vi "test notifier.vi"() -> ()   [LabVIEW 2019]
uses:
  Controls/FGV States.ctl
panel:
  in  "stop":bool
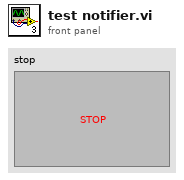
[diagram p1: front panel]
types:
  T1 = typedef "FGV States.ctl" = enum16{"Read", "Write"}
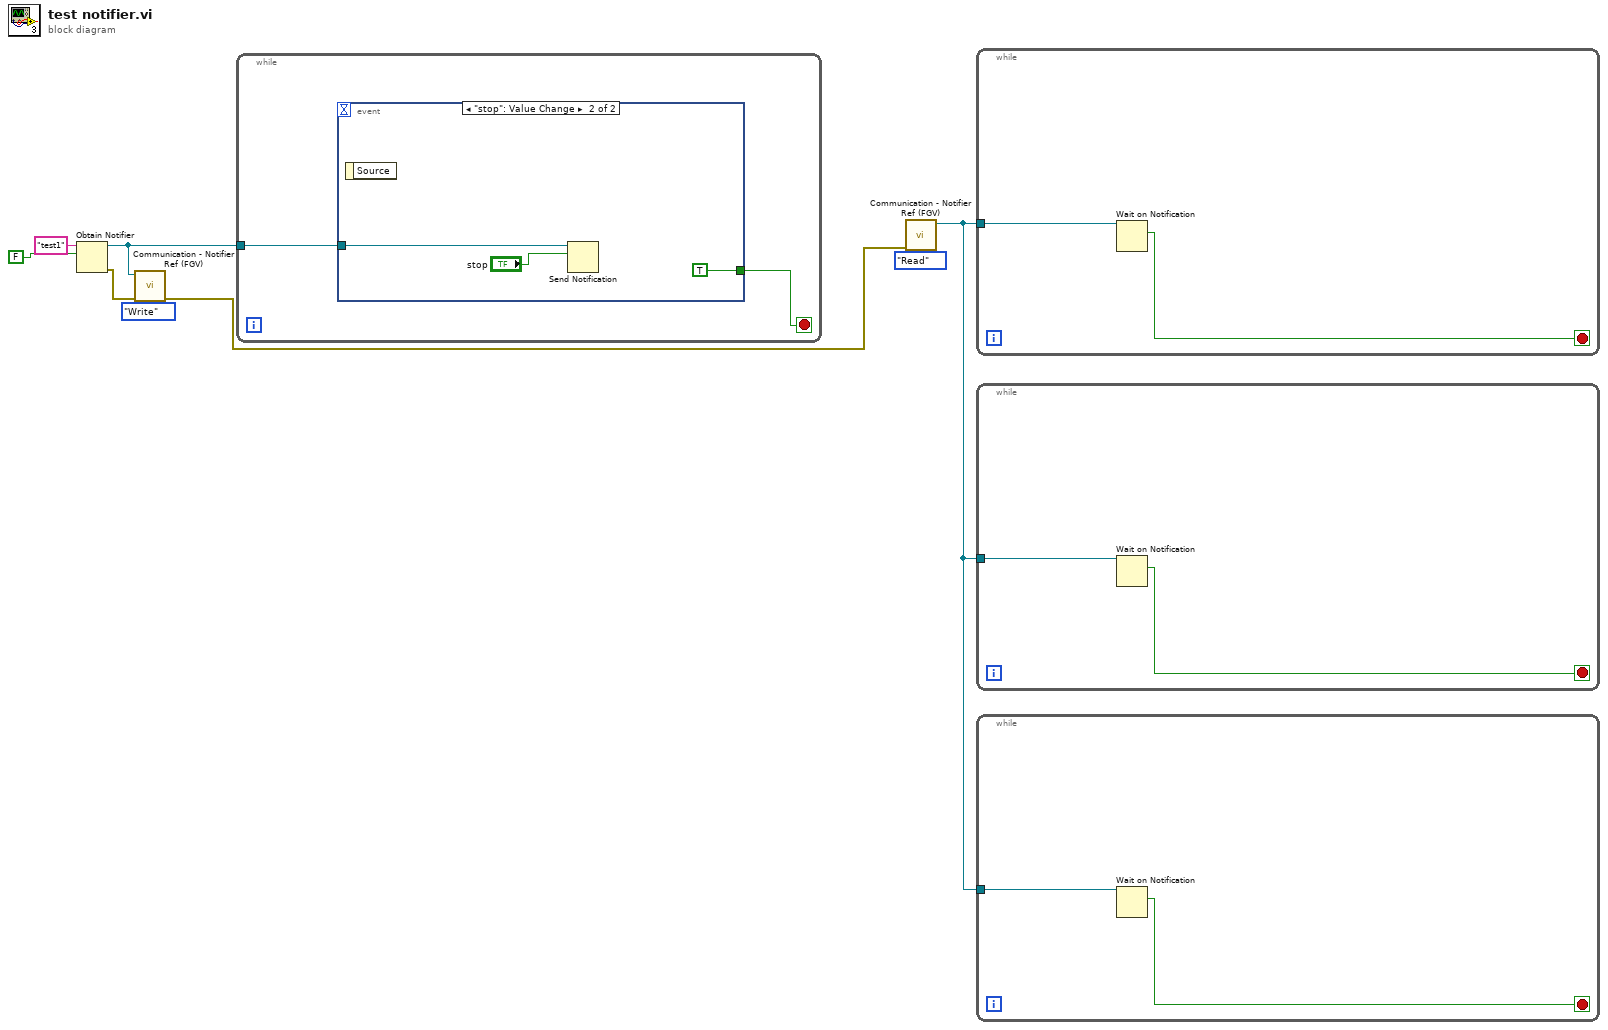
[diagram p0: block diagram]
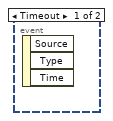
[diagram p2: hidden frame]
diagram:
  n1 = Obtain Notifier(name (unnamed)="test1", notification data type=FALSE) -> (notifier out=w6:refnum<notifier>, error out=w4:errorcluster)  [unwired: 2 in, 1 out]
  n2 = call "Communication - Notifier Ref (FGV).vi"("Action"=FGV_States."Write", "error in (no error)"=w4, "notifier in"=w6) -> ("error out"=w2:errorcluster)  [unwired: 7 in, 1 out]
  n3 = while {
    tunnel: w6 -> [w10]
    stop <- w9 stop-if-true
    n4 = event shown="[1] \"stop\": Value Change" {
      selector: _ -> [_ _]
      dyn-events: _ -> [_ _]
      timeout: _ -> [_ _]
      tunnel: w10 -> [_ w12]
      tunnel: [_ TRUE] -> w9
      event Timeout {
        n5 = event-data() -> ()  [unwired: 1 in, 3 out]
      }
      event "stop": Value Change {
        n6 = event-data() -> ()  [unwired: 1 in, 1 out]
        n7 = Send Notification(notification="stop", notifier=w12) -> ()  [unwired: 1 in, 2 out]
      }
    }
  }
  n8 = call "Communication - Notifier Ref (FGV).vi"("Action"=FGV_States."Read", "error in (no error)"=w2) -> ("notifier out"=w1:refnum<notifier>)  [unwired: 8 in, 1 out]
  n9 = while {
    tunnel: w1 -> [w15]
    stop <- w14 stop-if-true
    n10 = Wait on Notification(notifier=w15) -> (notification=w14:bool)  [unwired: 3 in, 3 out]
  }
  n11 = while {
    tunnel: w1 -> [w17]
    stop <- w16 stop-if-true
    n12 = Wait on Notification(notifier=w17) -> (notification=w16:bool)  [unwired: 3 in, 3 out]
  }
  n13 = while {
    tunnel: w1 -> [w19]
    stop <- w18 stop-if-true
    n14 = Wait on Notification(notifier=w19) -> (notification=w18:bool)  [unwired: 3 in, 3 out]
  }
